vi "Start.vi"(8 "error in (no error)":errorcluster, 11 "UDPlog Transceiver in":refnum<class "UDPlog Transceiver.lvclass">) -> (0 "error out":errorcluster, 3 "UDPlog Transceiver out":refnum<class "UDPlog Transceiver.lvclass">)   [LabVIEW 2023, in "UDPlog.lvlib" / "UDPlog Transceiver.lvclass"]
uses:
  UDPlog Transceiver.lvclass
  <vilib>/AddOns/VeriStand Custom Device Scripting APIs/Data Sharing Framework/DSF Core.lvlibp/Classes/Transceiver/Transceiver.lvclass
  UDPlog Transceiver.lvclass/UDPlog Transceiver.ctl
  <vilib>/Utility/SystemLogging/NI_SystemLogging.lvlib
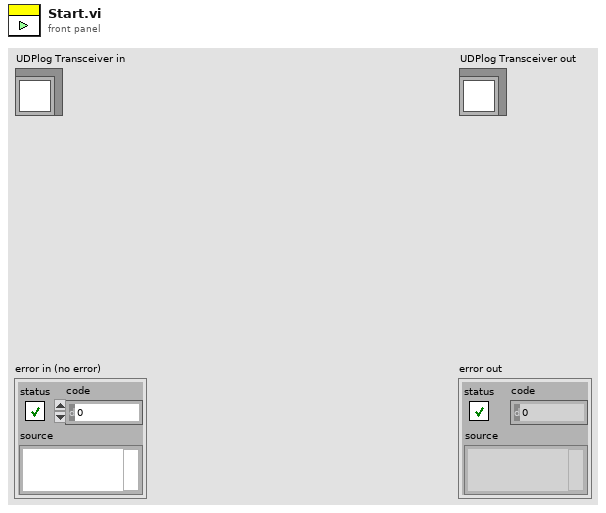
[diagram p1: front panel]
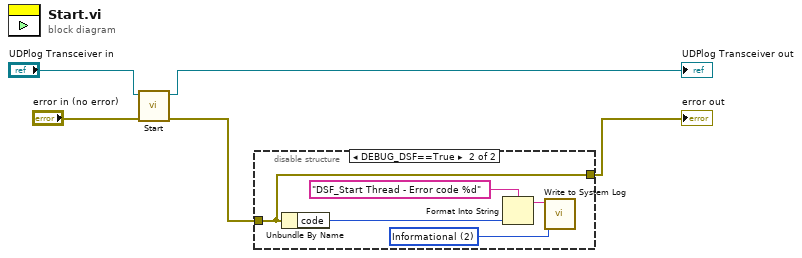
[diagram p0: block diagram]
diagram:
  n1 = call-parent "Start.vi"("error in (no error)"="error in (no error)", "Transceiver in"="UDPlog Transceiver in") -> ("error out"=w2:errorcluster, "Transceiver out"=→"UDPlog Transceiver out":refnum<class "UDPlog Transceiver.lvclass">)  [unwired: 8 in]
  n2 = disable-structure shown="DEBUG_DSF==True" {
    disable-tunnel: w2 -> [_ w8]
    disable-tunnel: [_ w8] -> w1
    frame condition #0 {
    }
    frame condition #1 (active) {
      w6 = 2 items=["Error", "Warning", "Informational"] ("severity")
      n3 = Unbundle By Name(w8) -> ("code"=w7:i32)
      n4 = Format Into String(format string="DSF_Start Thread - Error code %d", w7) -> (resulting string=w9:string)  [unwired: 2 in, 1 out]
      n5 = call <vilib>:"Write to System Log.vi"("severity"=w6, "message"=w9) -> ()  [unwired: 9 in, 1 out]
    }
  }
  "error out" <- w1
